vi "Examen01.vi"() -> ()   [LabVIEW 2020]
uses:
  <vilib>/numeric/Random Number (Range) U64.vi
  <vilib>/numeric/sub_Random U32.vi
panel:
  out "Datos guardados":bool caption="Saving Data"
  out "cantidad de numeros \ndentro del rango":dbl
  out "cantidad de numeros \nmayores al máximo":dbl
  out "Histerisis":bool
  in  "Maximo":u64
  in  "Minimo":u64
  out "Valor actual sin filtro":u64
  out "Grafica de datos aleatorios":cluster{dbl, dbl}(graph)
  in  "Guardar datos y\nterminar simulación":bool
  # "Valores para\nhisterisis"
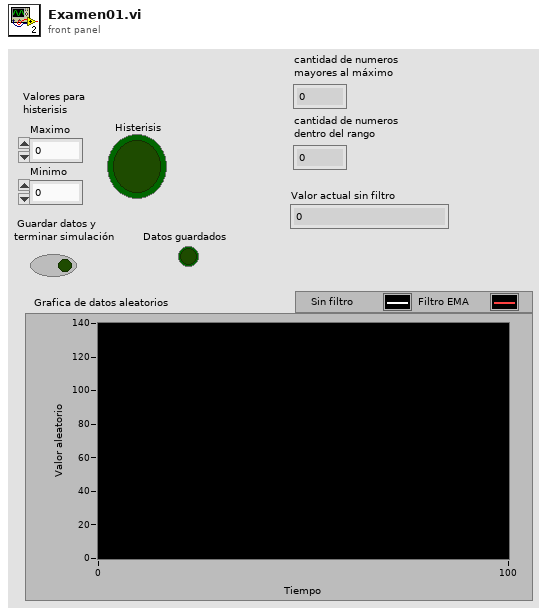
[diagram p1: front panel]
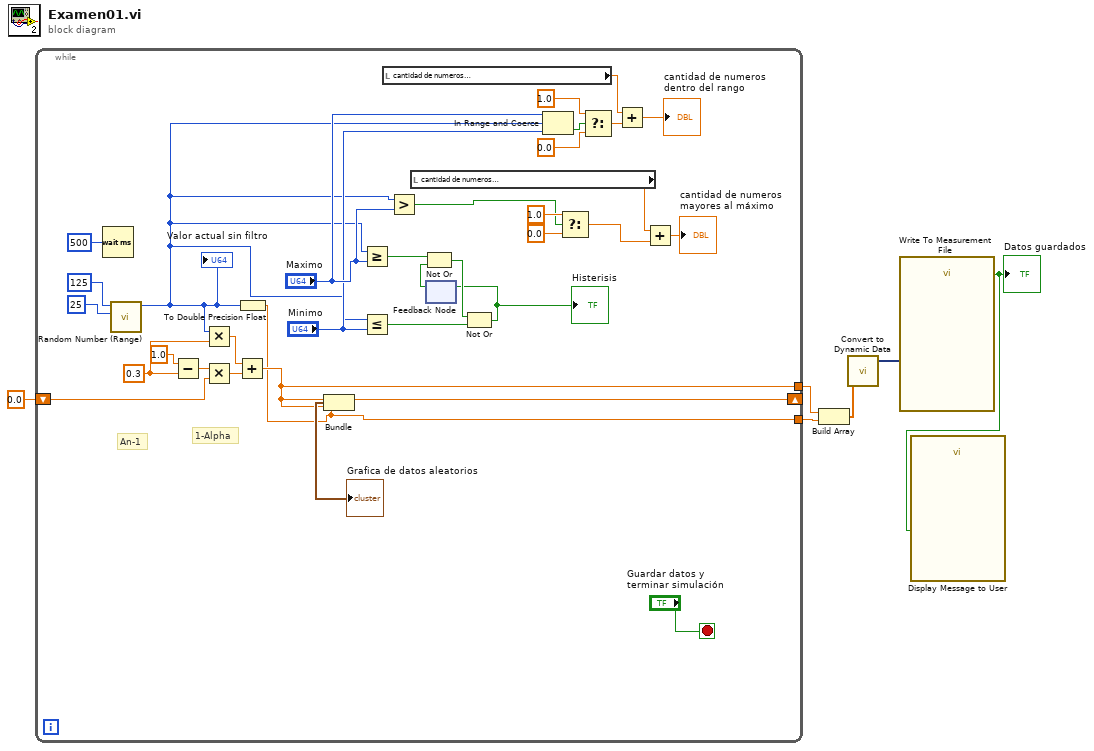
[diagram p0: block diagram]
diagram:
  n1 = while {
    shift-right: [w11] -> _
    shift-left: 0.0 -> [w32]
    tunnel: [w11] -> w5
    tunnel: [w10] -> w1
    stop <- "Guardar datos y\nterminar simulación" stop-if-true
    w31 = 0.3 ("Alpha")
    # "An-1"
    # "1-Alpha"
    n2 = Wait (ms)(milliseconds to wait=u32 500) -> ()  [unwired: 1 out]
    n3 = call-poly <vilib>:"Random Number (Range).vi"("lower bound (0)"=u64 25, "upper bound (100)"=u64 125) -> ("number"=w7:u64)  [unwired: 9 in]
    "Valor actual sin filtro" <- w7
    n4 = Subtract(x=1.0, y=w31) -> (x-y=w35:dbl)
    n5 = Multiply(x=w7, y=w31) -> (x*y=w34:dbl)
    n6 = Multiply(x=w35, y=w32) -> (x*y=w33:dbl)
    n7 = Add(x=w34, y=w33) -> (x+y=w11:dbl)
    n8 = To Double Precision Float(number=w7) -> (double precision float=w10:dbl)
    n9 = Bundle(w10, w11) -> (→"Grafica de datos aleatorios":cluster{dbl, dbl})  [unwired: 1 in]
    n10 = Greater Or Equal?(x=w7, y="Maximo") -> (x >= y?=w29:bool)
    n11 = Less Or Equal?(x=w7, y="Minimo") -> (x <= y?=w28:bool)
    n12 = local read "cantidad de numeros \ndentro del rango"() -> (w16:dbl)
    n13 = Greater?(x=w7, y="Maximo") -> (0:w20:bool)
    n14 = local read "cantidad de numeros \nmayores al máximo"() -> (w23:dbl)
    n15 = feedback #1() -> (w26:bool)  [unwired: 1 in]
    n16 = Not Or(1:w26, 2:w29) -> (0:w27:bool)
    n17 = Not Or(1:w28, 2:w27) -> (0:w21:bool)
    "Histerisis" <- w21
    n18 = feedback-in #1(w21) -> ()
    n19 = In Range and Coerce(upper limit="Maximo", x=w7, lower limit="Minimo") -> (In Range?=w17:bool)  [unwired: 1 out]
    n20 = Select(t=1.0, s=w20, f=0.0) -> (s? t:f=w22:dbl)
    n21 = Select(t=1.0, s=w17, f=0.0) -> (s? t:f=w15:dbl)
    n22 = Add(x=w16, y=w15) -> (x+y=→"cantidad de numeros \ndentro del rango":dbl)
    n23 = Add(x=w23, y=w22) -> (x+y=→"cantidad de numeros \nmayores al máximo":dbl)
  }
  n24 = Build Array(w5, w1) -> (w3:dbl[])
  n25 = call "Convert to Dynamic Data"("Array"=w3) -> ("Dynamic Data Type"=w2:dynamicdata)  [unwired: 3 in]
  n26 = call "Write To Measurement File"("Signals"=w2) -> ("Saving Data"=w4:bool)  [unwired: 16 in, 2 out]
  "Datos guardados" <- w4
  n27 = call "Display Message to User"("Enable"=w4) -> ()  [unwired: 9 in, 2 out]
